vi "Diag. Scale to Corridor.vi"(8 "Command Info In":T2, 10 "Block Inputs":T1={"Scale Angle"=38.0, "Distance"=18.0, "Speed"=0.75, "Corridor Angle"=0.0, "Elevator Height"=0.0}, 11 "Starting Position":T5) -> (0 "Command Info Out":T2)   [LabVIEW 2017]
uses:
  <vilib>/Rock Robotics/WPI/Framework/Command Status Info.ctl
  <vilib>/Rock Robotics/WPI/Framework/Completion Status.ctl
  <vilib>/Rock Robotics/WPI/Framework/Completion Notifier.ctl
  Support Code/Starting Position.ctl
  Block Clusters/Diag Scale to Corridor.ctl
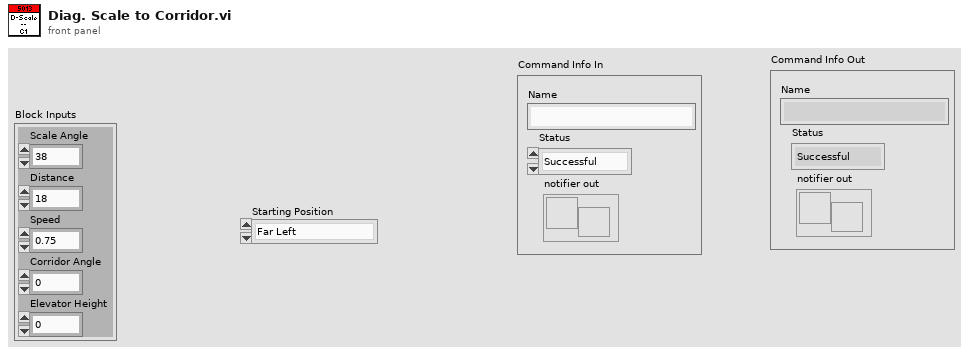
[diagram p1: front panel]
types:
  T1 = typedef "Diag Scale to Corridor.ctl" = cluster{"Scale Angle":dbl, "Distance":dbl, "Speed":dbl, "Corridor Angle":dbl, "Elevator Height":dbl}
  T2 = typedef "Command Status Info.ctl" = cluster{"Name":string, "Status":T3, "notifier out":T4}
  T3 = typedef "Completion Status.ctl" = enum16{"Successful", "Aborted", "Incomplete"}
  T4 = typedef "Completion Notifier.ctl" = refnum<notifier>
  T5 = typedef "Starting Position.ctl" = enum16{"Far Left", "Center", "Far Right"}
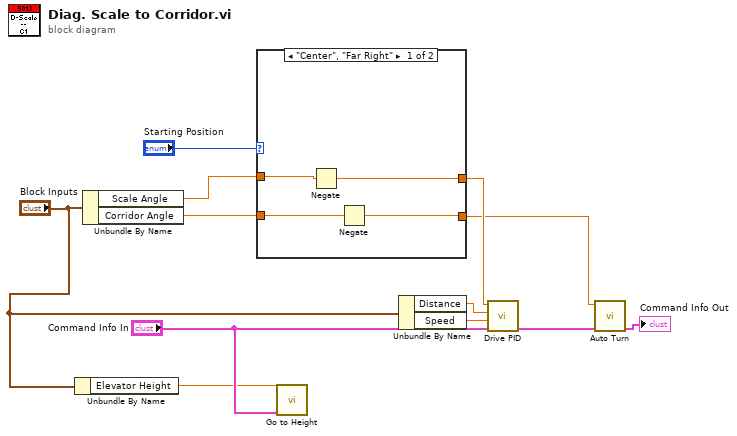
[diagram p0: block diagram]
diagram:
  n1 = Unbundle By Name("Block Inputs") -> ("Elevator Height"=w1:dbl)
  n2 = Unbundle By Name("Block Inputs") -> ("Scale Angle"=w10:dbl, "Corridor Angle"=w7:dbl)
  n3 = case shown="\"Center\", \"Far Right\"" "Starting Position" {
    tunnel: w10 -> [w16 w18]
    tunnel: [w15 w18] -> w9
    tunnel: [w13 w17] -> w8
    tunnel: w7 -> [w14 w17]
    frame "Center", "Far Right" {
      n4 = Negate(x=w16) -> (-x=w15:dbl)
      n5 = Negate(x=w14) -> (-x=w13:dbl)
    }
    frame "Far Left", Default {
    }
  }
  n6 = call "Go to Height.vi"("Command Info In"="Command Info In", "Target Height (in)"=w1) -> ()  [unwired: 9 in, 1 out]
  n7 = Unbundle By Name("Block Inputs") -> ("Distance"=w5:dbl, "Speed"=w6:dbl)
  n8 = call "Drive PID.vi"("Command Info In"="Command Info In", "Speed"=w6, "Distance"=w5, "Target Angle"=w9) -> ("Command Info Out"=w11:T2)  [unwired: 7 in]
  n9 = call "Auto Turn.vi"("Command Info In"=w11, "Target Angle"=w8) -> ("Command Info Out"=→"Command Info Out":T2)  [unwired: 9 in]
